vi "模式一.vi"() -> ()   [LabVIEW 2014]
panel:
  out "說明":string="本專題參考常見高中物理題型以及HW4。\n有一架轟炸機與一汽車水平距離為S0，轟炸機距離地面維持高度H並保持固定速度Va水平飛行，汽車速度固定為Vc，請問轟炸機飛行多久後投彈可以命中汽車?Va、Vc、S0、H皆為變數，重力加速度為9.81，本程式會將時間點算出，並以動態圖示意。"
  in  "stop":bool
  in  "OK Button":bool
  out "投彈時間(k)":dbl=2.0
  in  "Va":dbl=120.0
  in  "Vc":dbl=30.0
  in  "H":dbl=122.5
  in  "S0":i32=630
  out "轟炸機":T1=TRUE
  out "String":string
  out "炸彈":T2=TRUE
  out "車車":T3=TRUE
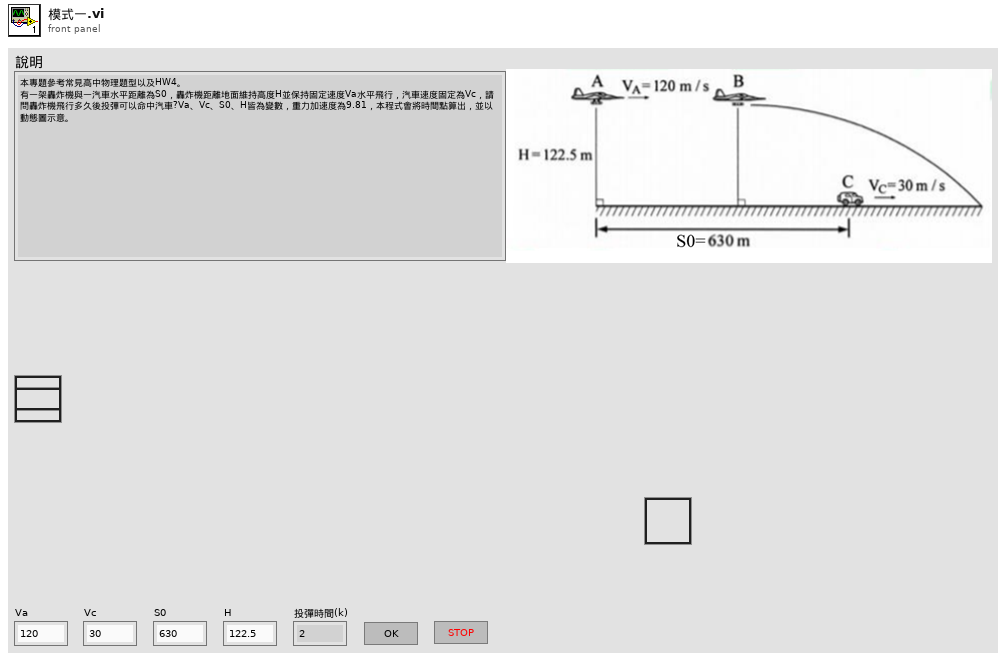
[diagram p1: front panel]
types:
  T1 = typedef "飛機.ctl" = bool
  T2 = typedef "炸彈.ctl" = bool
  T3 = typedef "車!!.ctl" = bool
  T4 = enum8{"Enabled", "Disabled", "Disabled and Grayed Out"}
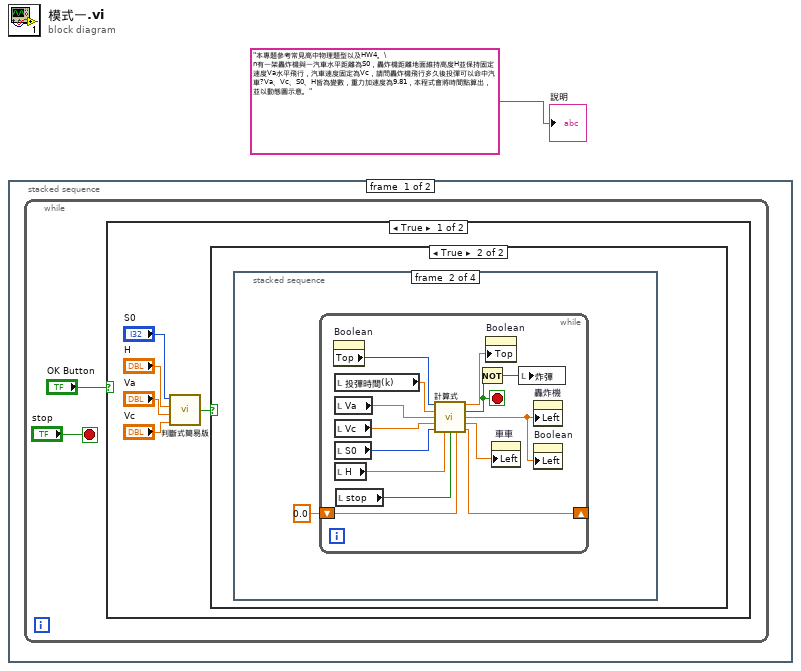
[diagram p0: block diagram]
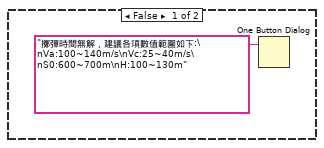
[diagram p2: hidden frame]
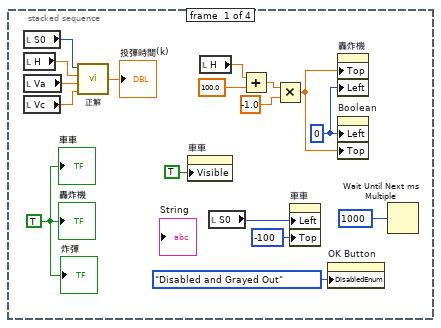
[diagram p3: hidden frame]
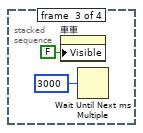
[diagram p4: hidden frame]
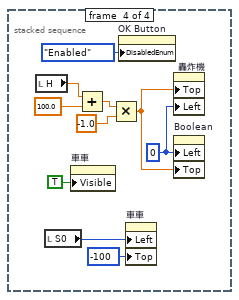
[diagram p5: hidden frame]
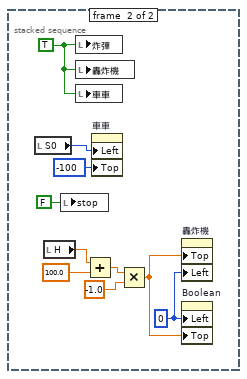
[diagram p7: hidden frame]
diagram:
  n1 = stacked-sequence {
    frame #0 {
      n2 = while {
        stop <- "stop" stop-if-true
        n3 = case shown="True" "OK Button" {
          frame True {
            n4 = call "判斷式簡易版.vi"("Vc"="Vc", "Va"="Va", "H"="H", "S0"="S0") -> ("result"=w4:bool)
            n5 = case shown="True" w4 {
              frame False {
                n6 = One Button Dialog(message="擲彈時間無解，建議各項數值範圍如下:\nVa:100~140m/s\nVc:25~40m/s\nS0:600~700m\nH:100~130m") -> ()  [unwired: 1 in, 1 out]
              }
              frame True {
                n7 = stacked-sequence {
                  frame #0 {
                    w21 = 0 ("Position:Left")
                    w24 = TRUE
                    n8 = local read "S0"() -> (w13:i32)
                    n9 = local read "H"() -> (w14:dbl)
                    n10 = local read "Va"() -> (w15:dbl)
                    n11 = local read "Vc"() -> (w16:dbl)
                    n12 = call "正解.vi"("Vc"=w16, "Va"=w15, "H"=w14, "S0"=w13) -> ("投彈時間(k)"=→"投彈時間(k)":dbl)
                    n13 = property on="車車" class="Bool (strict)"("Visible"=TRUE ("Caption.Visible")) -> ()  [unwired: 2 in, 2 out]
                    n14 = local read "H"() -> (w18:dbl)
                    n15 = local read "S0"() -> (w19:i32)
                    n16 = Add(x=w18, y=100.0) -> (x+y=w26:dbl)
                    n17 = Multiply(x=w26, y=-1.0) -> (x*y=w22:dbl)
                    n18 = property on="車車" class="Bool (strict)"("Left"=w19, "Top"=-100 ("Position:Top")) -> ()  [unwired: 2 in, 2 out]
                    n19 = property on="OK Button" class="Bool"("DisabledEnum"=T4."Disabled and Grayed Out" ("Disabled")) -> ()  [unwired: 2 in, 2 out]
                    n20 = property on="轟炸機" class="Bool (strict)"("Top"=w22, "Left"=w21) -> ()  [unwired: 2 in, 2 out]
                    n21 = property on="Boolean" class="Bool (strict)"("Left"=w21, "Top"=w22) -> ()  [unwired: 2 in, 2 out]
                    n22 = Wait Until Next ms Multiple(millisecond multiple=u32 1000) -> ()  [unwired: 1 out]
                    "車車" <- w24
                    "轟炸機" <- w24
                    "炸彈" <- w24
                  }
                  frame #1 {
                    n23 = while {
                      shift-right: [w30] -> _
                      shift-left: 0.0 -> [w34]
                      stop <- w29 stop-if-true
                      n24 = property on="Boolean" class="Bool (strict)"() -> ("Top"=w41:i32)  [unwired: 2 in, 2 out]
                      n25 = local read "投彈時間(k)"() -> (w40:dbl)
                      n26 = local read "Va"() -> (w39:dbl)
                      n27 = local read "Vc"() -> (w38:dbl)
                      n28 = local read "S0"() -> (w37:i32)
                      n29 = local read "H"() -> (w36:dbl)
                      n30 = local read "stop"() -> (w35:bool)
                      n31 = call "計算式.vi"("b y"=w41, "投彈時間(k)"=w40, "Va"=w39, "Vc"=w38, "S0"=w37, "H"=w36, "stop"=w35, "ti"=w34) -> ("b y 2"=w33:dbl, "output stop"=w29:bool, "a x"=w32:dbl, "c x"=w31:dbl, "to"=w30:dbl)  [unwired: 3 in]
                      n32 = Not(x=w29) -> (.not. x?=w28:bool)
                      n33 = property on="Boolean" class="Bool (strict)"("Top"=w33) -> ()  [unwired: 2 in, 2 out]
                      n34 = property on="車車" class="Bool (strict)"("Left"=w31) -> ()  [unwired: 2 in, 2 out]
                      n35 = local write "炸彈"(w28) -> ()
                      n36 = property on="轟炸機" class="Bool (strict)"("Left"=w32) -> ()  [unwired: 2 in, 2 out]
                      n37 = property on="Boolean" class="Bool (strict)"("Left"=w32) -> ()  [unwired: 2 in, 2 out]
                    }
                  }
                  frame #2 {
                    n38 = property on="車車" class="Bool (strict)"("Visible"=FALSE ("Caption.Visible")) -> ()  [unwired: 2 in, 2 out]
                    n39 = Wait Until Next ms Multiple(millisecond multiple=u32 3000) -> ()  [unwired: 1 out]
                  }
                  frame #3 {
                    w48 = 0 ("Position:Left")
                    n40 = local read "H"() -> (w45:dbl)
                    n41 = local read "S0"() -> (w46:i32)
                    n42 = property on="車車" class="Bool (strict)"("Visible"=TRUE ("Caption.Visible")) -> ()  [unwired: 2 in, 2 out]
                    n43 = Add(x=w45, y=100.0) -> (x+y=w52:dbl)
                    n44 = Multiply(x=w52, y=-1.0) -> (x*y=w49:dbl)
                    n45 = property on="OK Button" class="Bool"("DisabledEnum"=T4."Enabled" ("Disabled")) -> ()  [unwired: 2 in, 2 out]
                    n46 = property on="車車" class="Bool (strict)"("Left"=w46, "Top"=-100 ("Position:Top")) -> ()  [unwired: 2 in, 2 out]
                    n47 = property on="轟炸機" class="Bool (strict)"("Top"=w49, "Left"=w48) -> ()  [unwired: 2 in, 2 out]
                    n48 = property on="Boolean" class="Bool (strict)"("Left"=w48, "Top"=w49) -> ()  [unwired: 2 in, 2 out]
                  }
                }
              }
            }
          }
          frame False {
          }
        }
      }
    }
    frame #1 {
      w59 = 0 ("Position:Left")
      w62 = TRUE
      n49 = local read "S0"() -> (w55:i32)
      n50 = local read "H"() -> (w61:dbl)
      n51 = local write "stop"(FALSE ("stop")) -> ()
      n52 = local write "炸彈"(w62) -> ()
      n53 = local write "轟炸機"(w62) -> ()
      n54 = local write "車車"(w62) -> ()
      n55 = Add(x=w61, y=100.0) -> (x+y=w56:dbl)
      n56 = property on="車車" class="Bool (strict)"("Left"=w55, "Top"=-100 ("Position:Top")) -> ()  [unwired: 2 in, 2 out]
      n57 = Multiply(x=w56, y=-1.0) -> (x*y=w58:dbl)
      n58 = property on="轟炸機" class="Bool (strict)"("Top"=w58, "Left"=w59) -> ()  [unwired: 2 in, 2 out]
      n59 = property on="Boolean" class="Bool (strict)"("Left"=w59, "Top"=w58) -> ()  [unwired: 2 in, 2 out]
    }
  }
  "說明" <- "本專題參考常見高中物理題型以及HW4。\n有一架轟炸機與一汽車水平距離為S0，轟炸機距離地面維持高度H並保持固定速度Va水平飛行，汽車速度固定為Vc，請問轟炸機飛行多久後投彈可以命中汽車?Va、Vc、S0、H皆為變數，重力加速度為9.81，本程式會將時間點算出，並以動態圖示意。" ("說明")
